vi "Two Button Dialog.vi"(8 "error in (no error)":errorcluster, 9 "Retry Text In":string, 10 "Cancel Text In":string, 11 "Message Text In":string) -> (0 "error out":errorcluster, 2 "Continue?":bool)   [LabVIEW 2020, in "UI.lvlib"]
uses:
  UI.lvlib
panel:
  out "Display String":string
  in  "Retry":bool
  in  "Cancel":bool
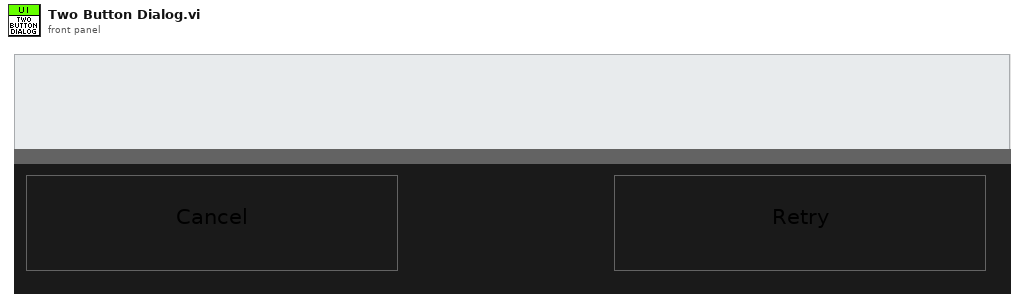
[diagram p1: front panel]
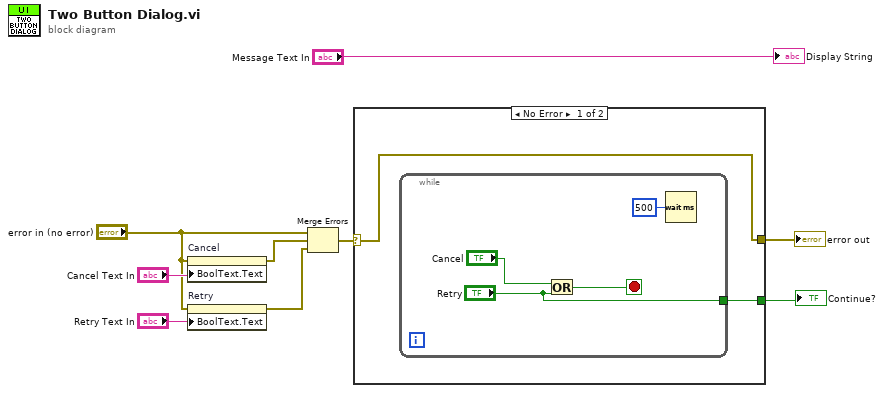
[diagram p0: block diagram]
diagram:
  n1 = property on="Cancel" class="Bool"(error in="error in (no error)", "BoolText.Text"="Cancel Text In") -> (error out=w5:errorcluster)  [unwired: 1 in, 1 out]
  n2 = property on="Retry" class="Bool"(error in="error in (no error)", "BoolText.Text"="Retry Text In") -> (error out=w4:errorcluster)  [unwired: 1 in, 1 out]
  n3 = Merge Errors("error in (no error)", w5, w4) -> (w6:errorcluster)
  n4 = case shown="No Error" w6 {
    selector: w6 -> [w10 w16]
    tunnel: [w11 _] -> w2
    tunnel: [w10 w16] -> w1
    frame No Error {
      n5 = while {
        tunnel: ["Retry"] -> w11
        stop <- w13 stop-if-true
        n6 = Or(x="Cancel", y="Retry") -> (x .or. y?=w13:bool)
        n7 = Wait (ms)(milliseconds to wait=u32 500) -> ()  [unwired: 1 out]
      }
    }
    frame Error {
    }
  }
  "error out" <- w1
  "Continue?" <- w2
  "Display String" <- "Message Text In"
